vi "Write Stack Light State.vi"(8 "error in (no error)":errorcluster, 9 "Light Mode":T2, 10 "Light Select":T1, 11 "DigitalIO in":refnum<class "DigitalIO.lvclass">) -> (0 "error out":errorcluster, 3 "DigitalIO out":refnum<class "DigitalIO.lvclass">)   [LabVIEW 2018, in "DigitalIO.lvlib" / "DigitalIO.lvclass"]
uses:
  DigitalIO.lvclass
  PPLs/PLC/Light Stack.lvlibp/Custom Controls/Light Mode.ctl
  PPLs/PLC/Light Stack.lvlibp/Custom Controls/Light Select.ctl
  DigitalIO.lvclass/DigitalIO.ctl
  PPLs/PLC/Light Stack.lvlibp/Light Stack.lvclass
  PPLs/PLC/Light Stack.lvlibp
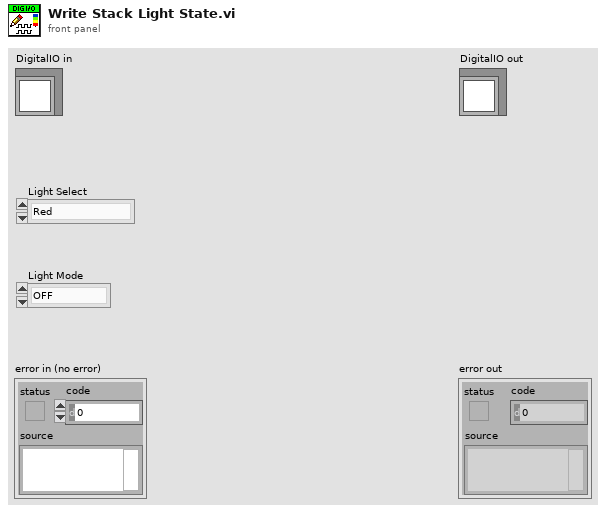
[diagram p1: front panel]
types:
  T1 = typedef "Light Stack.lvlibp/Light Select.ctl" = enum16{"Red", "Amber", "Green", "Blue"}
  T2 = typedef "Light Stack.lvlibp/Light Mode.ctl" = enum16{"OFF", "ON", "BLINK"}
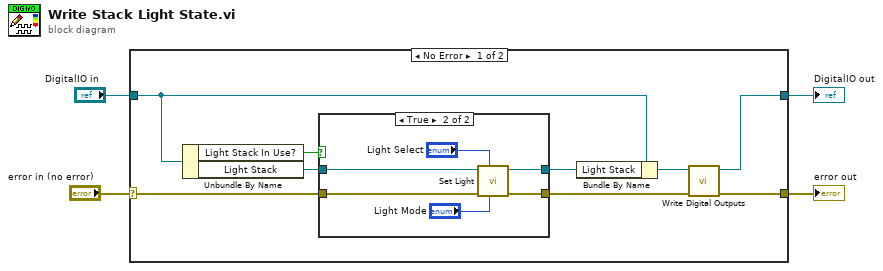
[diagram p0: block diagram]
diagram:
  n1 = case shown="No Error" "error in (no error)" {
    selector: "error in (no error)" -> [w11 w23]
    tunnel: [w5 w23] -> w3
    tunnel: [w6 w22] -> w1
    tunnel: "DigitalIO in" -> [w10 w22]
    frame No Error {
      n2 = Unbundle By Name(w10) -> ("Light Stack In Use?"=w13:bool, "Light Stack"=w12:refnum<class "Light Stack.lvclass">)
      n3 = case shown="True" w13 {
        tunnel: w12 -> [w15 w21]
        tunnel: w11 -> [w14 w18]
        tunnel: [w14 w17] -> w7
        tunnel: [w15 w16] -> w9
        frame False {
        }
        frame True {
          n4 = call "Set Light.vi"("State"="Light Mode", "Light Select"="Light Select", "error in"=w18, "Light Stack in"=w21) -> ("error out"=w17:errorcluster, "Light Stack out"=w16:refnum<class "Light Stack.lvclass">)  [unwired: 6 in]
        }
      }
      n5 = Bundle By Name(cluster=w10, "Light Stack"=w9) -> (w8:refnum<class "DigitalIO.lvclass">)
      n6 = call-dynamic "Write Digital Outputs.vi"("error in (no error)"=w7, "DigitalIO in"=w8) -> ("error out"=w5:errorcluster, "DigitalIO out"=w6:refnum<class "DigitalIO.lvclass">)  [unwired: 8 in]
    }
    frame Error {
    }
  }
  "error out" <- w3
  "DigitalIO out" <- w1
